vi "Position Back Button.vi"(8 "error in (no error)":errorcluster, 10 "Previous Button Refnum":refnum<vi>, 11 "Bool Refnum":refnum<vi>) -> (0 "error out":errorcluster)   [LabVIEW 2014]
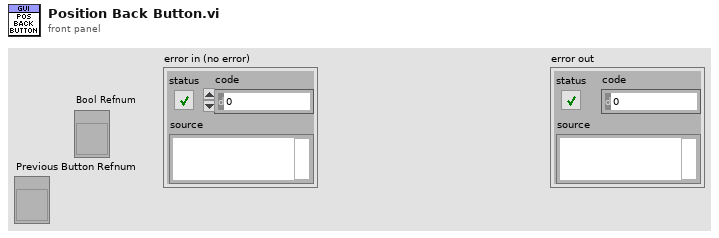
[diagram p1: front panel]
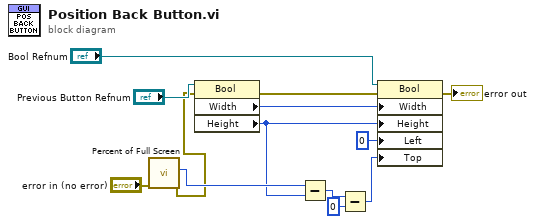
[diagram p0: block diagram]
diagram:
  n1 = call "Percent of Full Screen.vi"("error in (no error)"="error in (no error)") -> ("error out"=w5:errorcluster, "Bottom"=w12:i16)  [unwired: 8 in, 1 out]
  n2 = property class="Bool"(reference="Previous Button Refnum", error in=w5) -> (error out=w9:errorcluster, "Width"=w8:u32, "Height"=w7:u32)  [unwired: 1 out]
  n3 = Subtract(x=w12, y=w7) -> (x-y=w3:u32)
  n4 = Subtract(x=w3, y=u32 0) -> (x-y=w1:u32)
  n5 = property class="Bool"(reference="Bool Refnum", error in=w9, "Width"=w8, "Height"=w7, "Left"=0 ("Position:Left"), "Top"=w1) -> (error out=→"error out":errorcluster)  [unwired: 1 out]
